vi "Distance_Between_pointes.vi"(1 "P2":dbl[](array[numeric])=[191.0, -700.0, 65.0], 2 "P1":dbl[](array[numeric])=[191.0, -700.0, 65.0]) -> (0 "Distance":dbl)   [LabVIEW 2010]
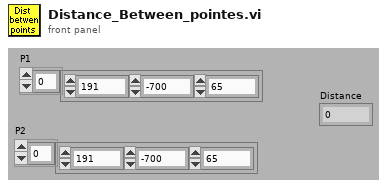
[diagram p1: front panel]
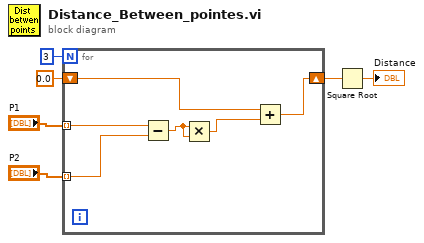
[diagram p0: block diagram]
diagram:
  n1 = for {
    N: 3 -> [_]
    tunnel: "P1" -> [w11] mode=indexing
    tunnel: "P2" -> [w10] mode=indexing
    shift-right: [w7] -> w3
    shift-left: 0.0 -> [w8]
    n2 = Subtract(x=w11, y=w10) -> (x-y=w12:dbl)
    n3 = Multiply(x=w12, y=w12) -> (x*y=w9:dbl)
    n4 = Add(x=w8, y=w9) -> (x+y=w7:dbl)
  }
  n5 = Square Root(x=w3) -> (sqrt(x)=→"Distance":dbl)
